vi "step_motor_pitch.vi"(6 "F_Threshold":fxp<+,12,12>, 10 "omega_p":fxp<+/-,20,9>, 11 "F":fxp<+/-,20,10>) -> (1 "vq_F":fxp<+/-,20,5> format="%.57g", 3 "vd_F":fxp<+/-,20,5>)   [LabVIEW 2014]
uses:
  <vilib>/rvi/FXPMathLib/FxpMul/XNode/nifxpmath_Multiplier.xnode
  <vilib>/rvi/FXPMathLib/FxpAdd/XNode/nifxpmath_Add.xnode
  <vilib>/rvi/FXPMathLib/sim/FxpSim.dll
panel:
  out "-RKm/NrL":fxp<+/-,18,2>=-1.9615478515625
  out "tauR/Km":fxp<+/-,30,15>
  out "Kmw":fxp<+/-,25,10> format="%.50g"
  out "-NrLwtau/Km":fxp<+/-,36,21> format="%.54g"
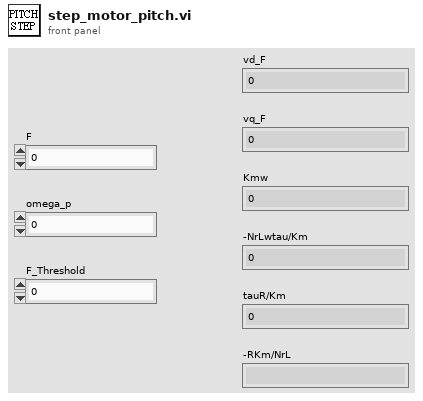
[diagram p1: front panel]
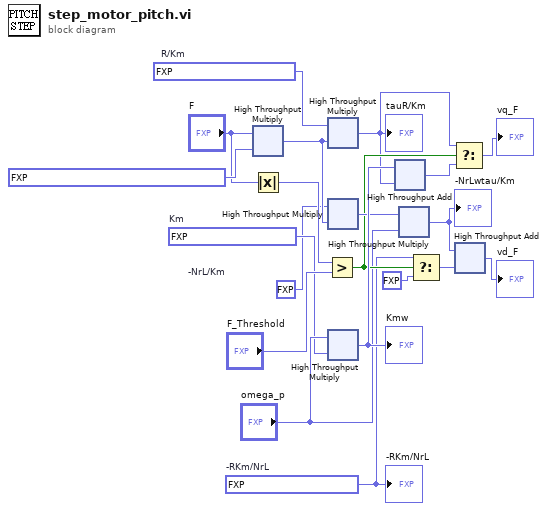
[diagram p0: block diagram]
diagram:
  w1 = fxp<+/-,20,4> -8.0  # -NrL/Km
  w2 = fxp<+/-,18,2> -0.9384002685546875  # -RKm/NrL
  w3 = fxp<+,23,7> 112.52980041503906  # R/Km
  w4 = fxp<+,14,-2> 0.0865325927734375  # Km
  n1 = xnode ("High Throughput Multiply")("x"="F", "y"=fxp<+/-,28,0> -0.0003853030502796173) -> ("x*y"=w17:fxp<+/-,15,-1>)
  n2 = Absolute Value(x="F") -> (abs(x)=w16:fxp<+,20,10>)
  n3 = Greater?(x=w16, y="F_Threshold") -> (0:w10:bool)
  n4 = xnode ("High Throughput Multiply")("x"=w3, "y"=w17) -> ("x*y"=w8:fxp<+/-,20,5>)
  "tauR/Km" <- w8
  n5 = xnode ("High Throughput Multiply")("x"=w1, "y"=w17) -> ("x*y"=w19:fxp<+/-,17,1>)
  n6 = xnode ("High Throughput Multiply")("x"="omega_p", "y"=w4) -> ("x*y"=w20:fxp<+/-,22,7>)
  "Kmw" <- w20
  n7 = xnode ("High Throughput Add")("x"=w20, "y"=w8) -> ("x+y"=w9:fxp<+/-,20,5>)
  n8 = xnode ("High Throughput Multiply")("x"=w19, "y"="omega_p") -> ("x*y"=w14:fxp<+/-,20,5>)
  "-NrLwtau/Km" <- w14
  n9 = Select(t=w2, s=w10, f=fxp<+/-,18,2> 0.0) -> (s? t:f=w12:fxp<+/-,18,2>)
  n10 = Select(t=w8, s=w10, f=w9) -> (s? t:f=→"vq_F":fxp<+/-,20,5>)
  n11 = xnode ("High Throughput Add")("x"=w14, "y"=w12) -> ("x+y"=→"vd_F":fxp<+/-,20,5>)
  "-RKm/NrL" <- w2
